vi "Pump Controller.vi"() -> ()   [LabVIEW 2024]
uses:
  Pump Switch.ctl
panel:
  in  "Pump State":T1
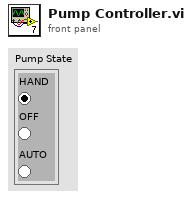
[diagram p1: front panel]
types:
  T1 = typedef "Pump Switch.ctl" = enum32{"HAND", "OFF", "AUTO"}
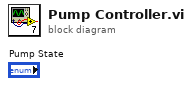
[diagram p0: block diagram]
diagram:
